vi "截取ROI图像.vi"(1 "ROI(T3)":T2, 2 "输入Image":T1) -> (0 "输出image数组":u8[][](array[numeric]))   [LabVIEW 2017]
uses:
  <vilib>/vision/Image Controls.llb/IMAQ Image.ctl
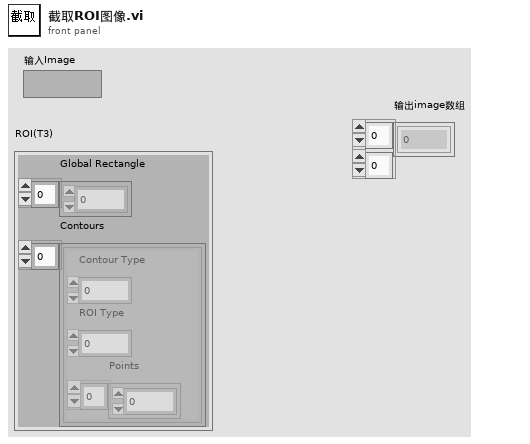
[diagram p1: front panel]
types:
  T1 = typedef "IMAQ Image.ctl" = refnum<image>
  T2 = cluster{"Global Rectangle":i32[], "Contours":cluster{"Contour Type":u32, "ROI Type":u32, "Points":i32[]}[]}
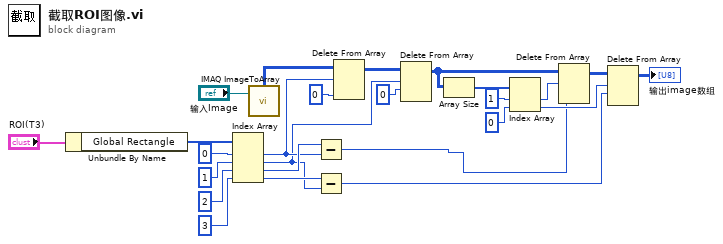
[diagram p0: block diagram]
diagram:
  n1 = Unbundle By Name("ROI(T3)") -> ("Global Rectangle"=w20:i32[])
  n2 = Index Array(array=w20, index #1=0, index #2=1, index #3=2, index #4=3) -> (element #1=w9:i32, element #2=w7:i32, element #3=w10:i32, element #4=w8:i32)
  n3 = call "IMAQ ImageToArray"("Image"="输入Image") -> ("Image Pixels (U8)"=w4:u8[][])  [unwired: 3 in, 4 out]
  n4 = Subtract(x=w10, y=w9) -> (x-y=w2:i32)
  n5 = Subtract(x=w8, y=w7) -> (x-y=w1:i32)
  n6 = Delete From Array(array=w4, length=w9, index (col)=0 ("禁用的索引 (列)")) -> (array with subset deleted=w18:u8[][])  [unwired: 1 in, 1 out]
  n7 = Delete From Array(array=w18, length=w7, index (row)=0 ("禁用的索引 (列)")) -> (array with subset deleted=w16:u8[][])  [unwired: 1 in, 1 out]
  n8 = Array Size(array=w16) -> (size(s)=w15:i32[])
  n9 = Index Array(array=w15, index #1=1 ("禁用的索引 (列)"), index #2=0) -> (element #1=w12:i32, element #2=w6:i32)
  n10 = Delete From Array(array=w16, length=w12, index (col)=w2) -> (array with subset deleted=w11:u8[][])  [unwired: 1 in, 1 out]
  n11 = Delete From Array(array=w11, length=w6, index (row)=w1) -> (array with subset deleted=→"输出image数组":u8[][])  [unwired: 1 in, 1 out]
